vi "Increment Counter.vi"(11 "Counter Data Plugin in":refnum<class "Counter Data Plugin.lvclass">) -> (2 "Counter":dbl, 3 "Counter Data Plugin out":refnum<class "Counter Data Plugin.lvclass">)   [LabVIEW 2017, in "Data Engine.lvlib" / "Counter Data Plugin.lvclass"]
uses:
  Counter Data Plugin.lvclass
  Counter Data Plugin.lvclass/Counter Data Plugin.ctl
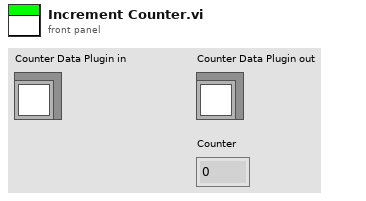
[diagram p1: front panel]
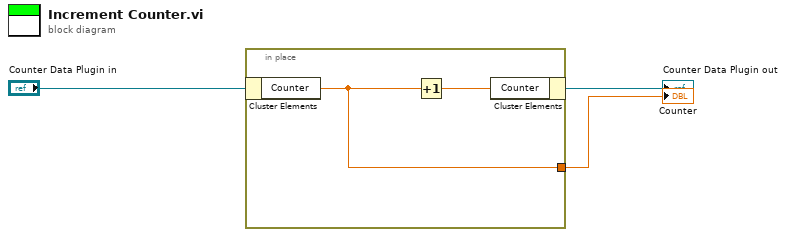
[diagram p0: block diagram]
diagram:
  n1 = in-place {
    in-place-border: [w4] -> w3
    n2 = in-place-cluster #1("Counter Data Plugin in") -> ("Counter"=w4:dbl)
    n3 = Increment(x=w4) -> (x+1=w5:dbl)
    n4 = in-place-cluster #1("Counter"=w5) -> (→"Counter Data Plugin out":refnum<class "Counter Data Plugin.lvclass">)
  }
  "Counter" <- w3
